vi "Bind Formatted String.vi"(4 "Ignore Past Updates? (F)":bool, 5 "Datum Type":variant, 6 "Format String":string, 8 "error in (no error)":errorcluster, 9 "Datum Name (\"\"=Use Control Label)":string, 10 "Str Refnum":refnum<vi>, 11 "IViewable in":refnum<class "IViewable.lvclass">) -> (0 "error out":errorcluster, 3 "IViewable out":refnum<class "IViewable.lvclass">)   [LabVIEW 2015, in "IViewable.lvlib" / "IViewable.lvclass"]
doc: "Bind a string control terminal (control or indicator) to a published value. You must provide a format string that is valid for the specified datum type."
uses:
  IViewable.lvclass
  <vilib>/ActorFramework/Actor/Actor.lvclass/Actor.ctl
  <vilib>/ActorFramework/Message Enqueuer/Message Enqueuer.lvclass/Message Enqueuer.ctl
  Transport/FormattedStringBinding/FormattedStringBinding.lvclass/FormattedStringBinding.ctl
  SubscriptionPolicy/ValueChangeSubscription/ValueChangeSubscription.lvclass/ValueChangeSubscription.ctl
  IMediator/SubscriptionRequest/SubscriptionRequest.lvclass/SubscriptionRequest.ctl
  IObserver/IObserver Messages/Subscribe Msg/Subscribe Msg.lvclass/Subscribe Msg.ctl
  <vilib>/ActorFramework/Message Enqueuer/Init from Existing Queue.vi
  <vilib>/ActorFramework/Message Enqueuer/Enqueue.vi
  <vilib>/ActorFramework/Message Priority Queue/Priority Enqueue.vi
  <vilib>/ActorFramework/Message Enqueuer/Message Enqueuer.lvclass
  Transport/FormattedStringBinding/FormattedStringBinding.lvclass
  SubscriptionPolicy/ValueChangeSubscription/ValueChangeSubscription.lvclass
  IMediator/SubscriptionRequest/SubscriptionRequest.lvclass
  IObserver/IObserver Messages/Subscribe Msg/Subscribe Msg.lvclass
  <vilib>/ActorFramework/Actor/Actor.lvclass
  IMediator/ISubscriptionPolicy/ISubscriptionPolicy.lvclass
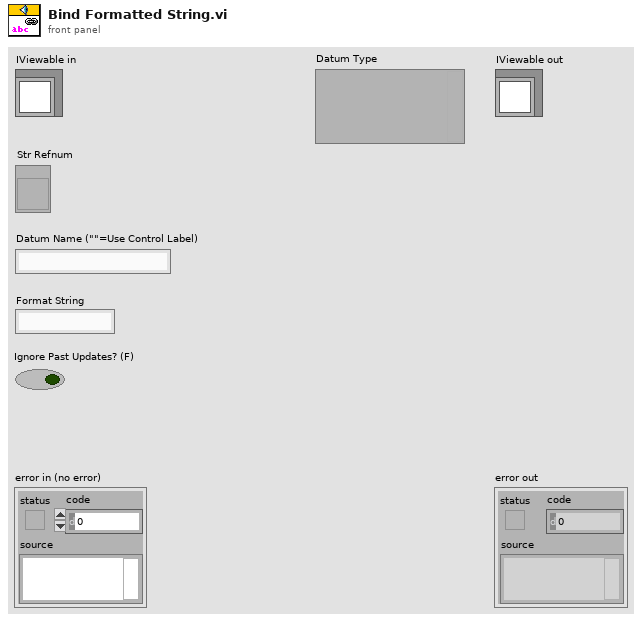
[diagram p1: front panel]
types:
  T1 = typedef "IMediator.lvlib/ISubscriptionPolicy.lvclass/ISubscriptionPolicy Reference.ctl" = refnum<data-value>
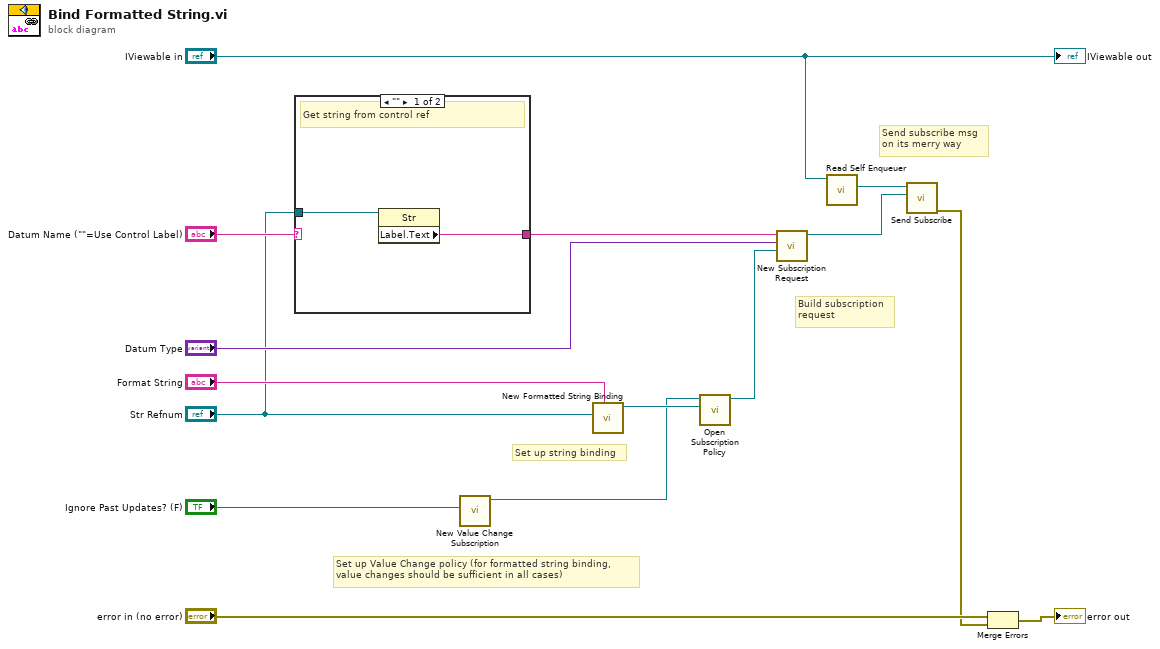
[diagram p0: block diagram]
diagram:
  # "Set up Value Change policy (for formatted string binding,\nvalue changes should be sufficient in all cases)"
  # "Send subscribe msg\non its merry way"
  # "Build subscription\nrequest"
  # "Set up string binding"
  n1 = case shown="\"\"" "Datum Name (\"\"=Use Control Label)" {
    selector: "Datum Name (\"\"=Use Control Label)" -> [_ w18]
    tunnel: [w16 w18] -> w9
    tunnel: "Str Refnum" -> [w17 _]
    frame "" {
      # "Get string from control ref"
      n2 = property class="Str"(reference=w17) -> ("Label.Text"=w16:string)  [unwired: 1 in, 2 out]
    }
    frame Default {
      # "Use string wired to input terminal"
    }
  }
  n3 = call "New Value Change Subscription.vi"("Ignore Past Updates? (F)"="Ignore Past Updates? (F)") -> ("ValueChangeSubscription Out"=w2:refnum<class "ValueChangeSubscription.lvclass">)  [unwired: 10 in]
  n4 = call "New Formatted String Binding.vi"("Format String"="Format String", "Str Refnum"="Str Refnum") -> ("FormattedStringBinding"=w5:refnum<class "FormattedStringBinding.lvclass">)  [unwired: 8 in, 1 out]
  n5 = call "Open Subscription Policy.vi"("Transport"=w5, "SubscriptionPolicy"=w2) -> ("Subscription Policy"=w1:T1)  [unwired: 8 in, 1 out]
  n6 = call "New Subscription Request.vi"("Subscription Policy"=w1, "Type"="Datum Type", "Datum Name"=w9) -> ("SubscriptionRequest"=w4:refnum<class "SubscriptionRequest.lvclass">)  [unwired: 8 in]
  n7 = call <vilib>:"Read Self Enqueuer.vi"("Actor"="IViewable in") -> ("Self Enqueuer"=w13:refnum<class "Message Enqueuer.lvclass">)  [unwired: 10 in]
  n8 = call "Send Subscribe.vi"("SubscriptionRequest"=w4, "Message Enqueuer"=w13) -> ("error out"=w11:errorcluster)  [unwired: 8 in, 1 out]
  n9 = Merge Errors("error in (no error)", w11) -> (→"error out":errorcluster)
  "IViewable out" <- "IViewable in"
